vi "Umgebung.ParameterUI.vi"() -> ()   [LabVIEW 2016, in "Umgebung.lvclass"]
uses:
  Umgebung.lvclass
  Package ResourceControl/ViHandler/ViHandler.ViInfo.ctl
  Package Libraries/Message Queue/private/MessageQueue.MessageTypeDef.ctl
  Umgebung.lvclass/Umgebung.ctl
  Package ErrorHandling/ErrorHandling.lvclass/ErrorHandling.ctl
  Read Umgebung.Parameter.vi
  Package ErrorHandling/ErrorHandling.checkForErrorAndHandle.vi
  Package ErrorHandling/ErrorHandling.GetErrorHandler.vi
  Package Libraries/StringFunctions/StringFunctions_ReplaceAllBlindSigns.vi
  <vilib>/dlg_ctls.llb/Space Constant.vi
  <vilib>/Utility/error.llb/Error Cluster From Error Code.vi
  Package Libraries/TimingFunctions/TimingFunctions_getUtcTimestamp.vi
  <vilib>/Utility/error.llb/Trim Whitespace.vi
  <vilib>/Utility/error.llb/Search and Replace Pattern.vi
  Package ErrorHandling/ErrorHandling.addLastErrorToFile.vi
  <vilib>/ErrorRing/Error Ring.xnode
  Package ErrorHandling/ErrorHandling.lvclass
  Package ResourceControl/ViHandler/ViHandler.lvclass
panel:
  in  "Umgebung Parameter":T1={"Wetter"=enum."Starke Bewölkung"}
  out "Umgebung":refnum<data-value>
  in  "Model Path":path
  out "ViInfoTemp":T2
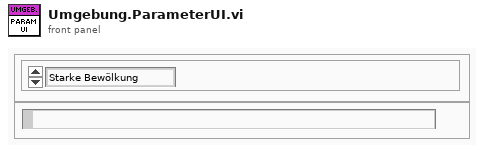
[diagram p1: front panel]
types:
  T1 = cluster{"Wetter":enum16{"Klarer Himmel", "Leichte Bewölkung", "Starke Bewölkung"}}
  T2 = typedef "ViHandler.lvclass/ViHandler.ViInfo.ctl" = cluster{"ViName":string, "ViReference":refnum<vi>, "ViQueueName":string}
  T3 = typedef "MessageQueue.MessageTypeDef.ctl" = cluster{"Message":string, "Data":variant}
  T4 = enum16{"open", "replace", "create", "open or create", "replace or create", "replace or create with confirmation"}
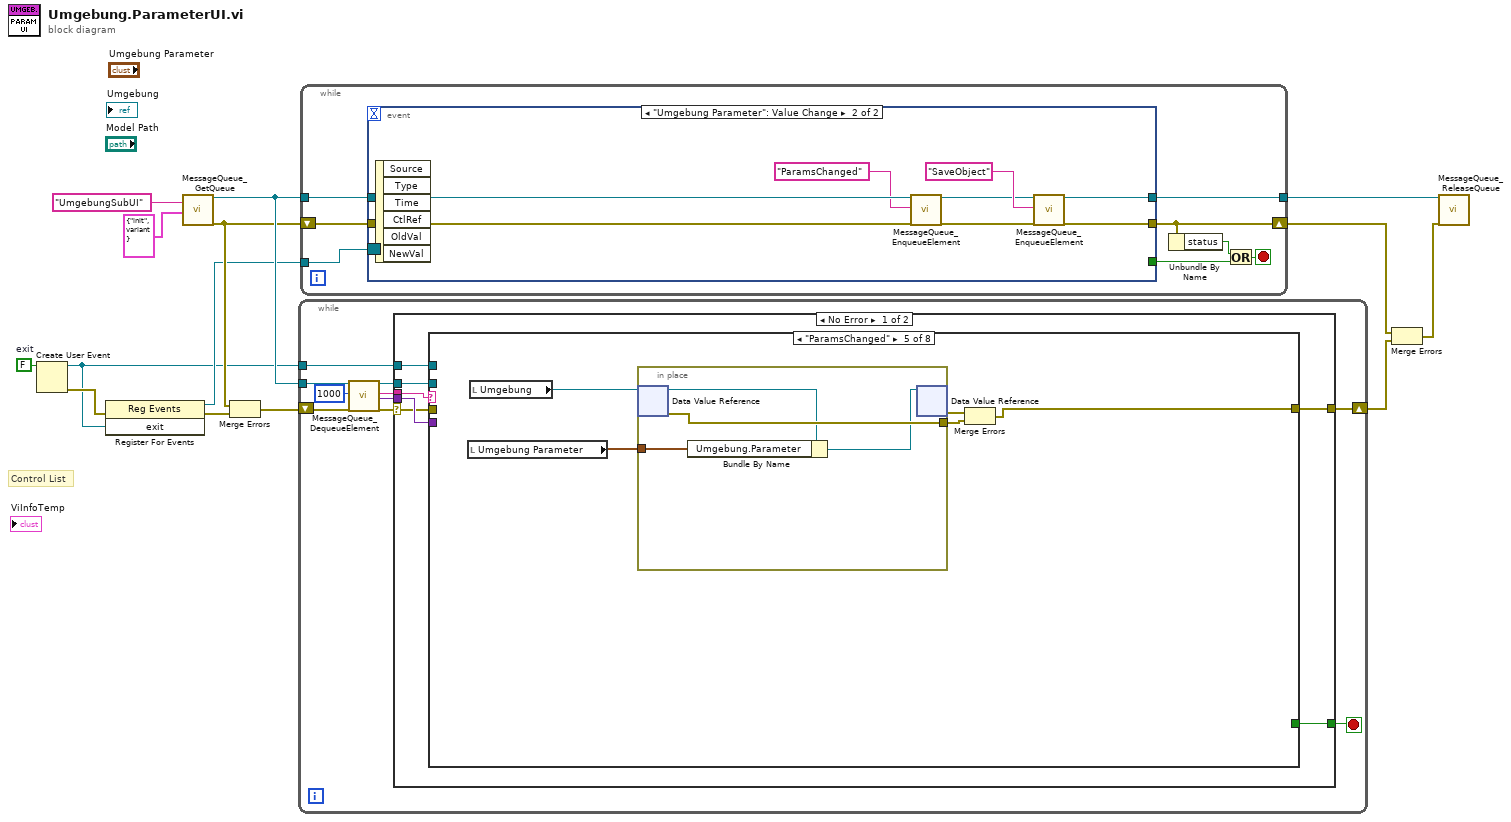
[diagram p0: block diagram]
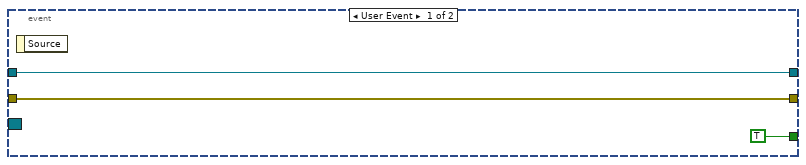
[diagram p2: hidden frame]
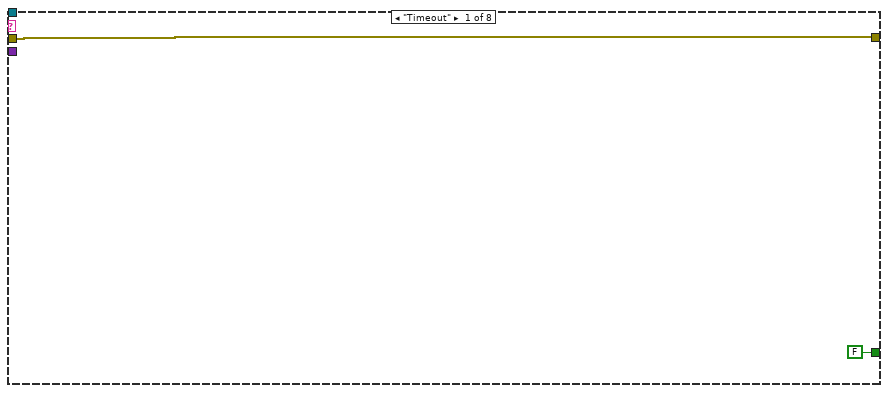
[diagram p3: hidden frame]
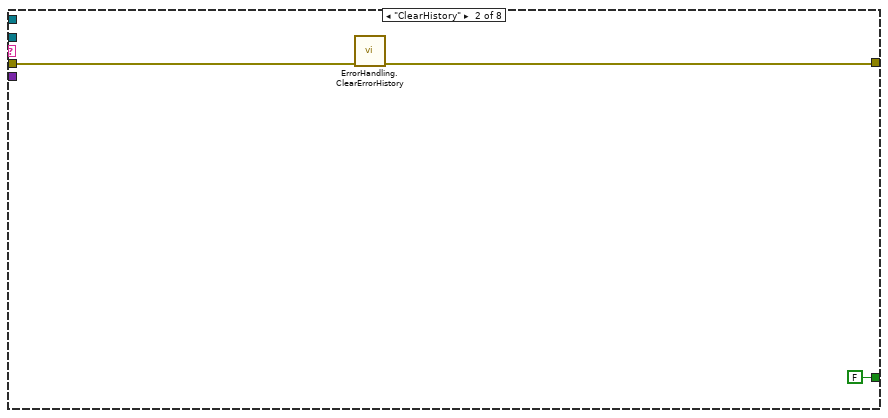
[diagram p4: hidden frame]
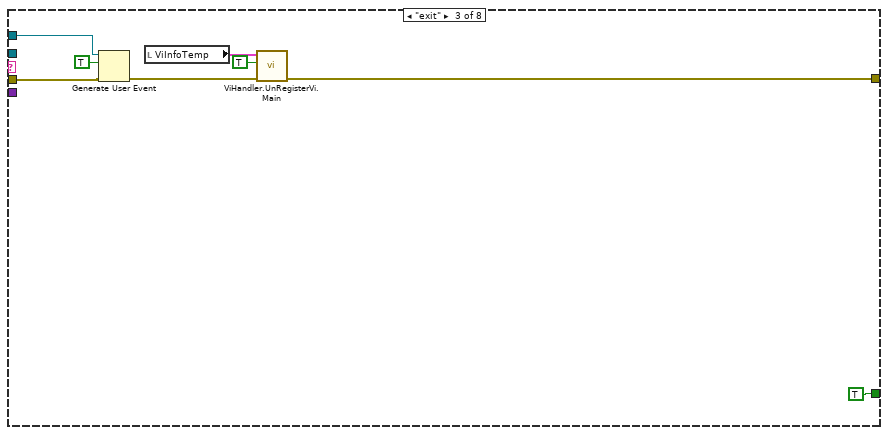
[diagram p5: hidden frame]
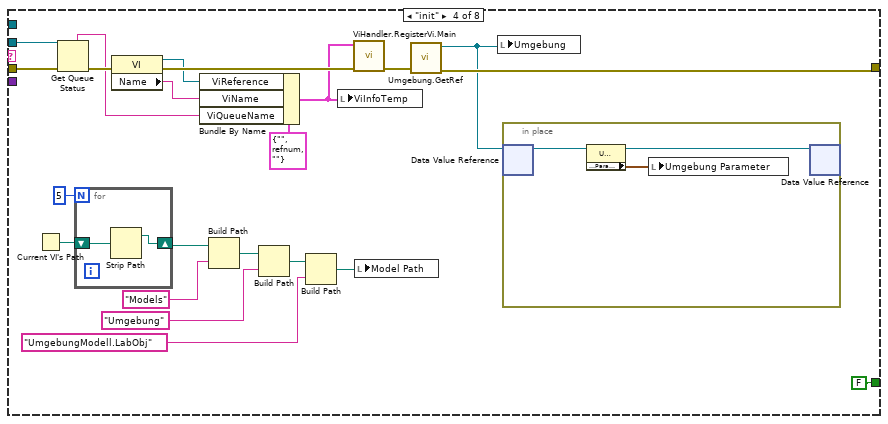
[diagram p6: hidden frame]
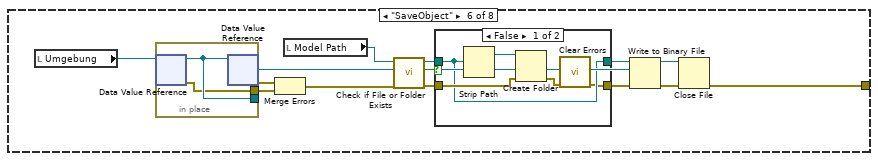
[diagram p7: hidden frame]
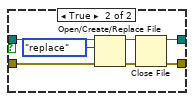
[diagram p8: hidden frame]
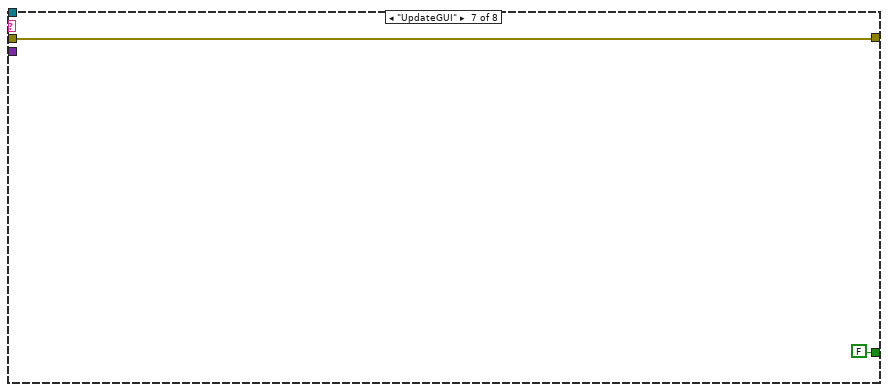
[diagram p9: hidden frame]
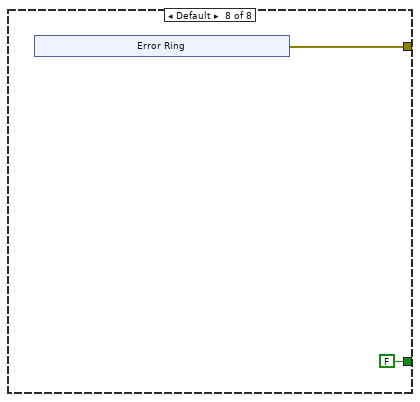
[diagram p10: hidden frame]
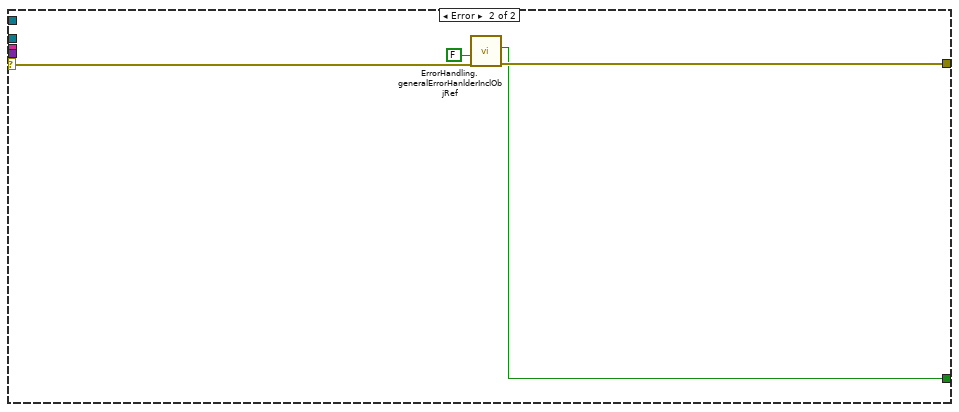
[diagram p11: hidden frame]
diagram:
  w7 = FALSE  # exit
  # "Control List"
  n1 = Create User Event(user event datatype=w7) -> (user event=w5:refnum<user-event>, error out=w6:errorcluster)  [unwired: 1 in]
  n2 = register-events(error in=w6, w5) -> (reference out=w9:refnum<event-registration>, error out=w11:errorcluster)  [unwired: 1 in]
  n3 = call "MessageQueue_GetQueue.vi"("Name"="UmgebungSubUI", "OptionalInitValue"=T3 {"Message"="init", "Data"=variant}) -> ("QueueOut"=w13:refnum<queue>, "ErrorOut"=w10:errorcluster)  [unwired: 15 in, 1 out]
  n4 = Merge Errors(w10, w11) -> (w8:errorcluster)
  n5 = while {
    tunnel: w13 -> [w24]
    tunnel: w5 -> [w17]
    shift-right: [w16] -> w3
    shift-left: w8 -> [w18]
    stop <- w19 stop-if-true
    n6 = call "MessageQueue_DequeueElement.vi"("QueueIn"=w24, "Timeout"=1000, "ErrorIn"=w18) -> ("QueueOut"=w22:refnum<queue>, "Message"=w21:string, "Data"=w20:variant, "ErrorOut"=w23:errorcluster)  [unwired: 12 in, 1 out]
    n7 = case shown="No Error" w23 {
      selector: w23 -> [w27 w121]
      tunnel: w22 -> [w31 _]
      tunnel: w21 -> [w30 _]
      tunnel: w20 -> [w29 _]
      tunnel: [w28 w119] -> w19
      tunnel: w17 -> [w26 _]
      tunnel: [w25 w120] -> w16
      frame No Error {
        n8 = case shown="\"ParamsChanged\"" w30 {
          tunnel: w31 -> [_ _ _ w60 _ _ _ _]
          tunnel: w29 -> [_ _ _ _ _ _ _ _]
          tunnel: [FALSE FALSE TRUE FALSE _ _ FALSE FALSE] -> w28
          tunnel: w27 -> [w32 w35 w42 w57 _ _ w109 _]
          tunnel: w26 -> [_ _ w41 _ _ _ _ _]
          tunnel: [w32 w34 w38 w46 w73 w82 w109 w112] -> w25
          frame "Timeout" {
          }
          frame "ClearHistory" {
            n9 = call "ErrorHandling.ClearErrorHistory.vi"("error IO"=w35) -> ("error IO"=w34:errorcluster)  [unwired: 10 in]
          }
          frame "exit" {
            n10 = Generate User Event(user event=w41, event data cluster=TRUE ("event data"), error in=w42) -> (error out=w39:errorcluster)  [unwired: 1 in, 1 out]
            n11 = local read "ViInfoTemp"() -> (w40:T2)
            n12 = call "ViHandler.UnRegisterVi.Main.vi"("ErrorIn"=w39, "FinalExit?"=TRUE, "ViInfo"=w40) -> ("ErrorOut"=w38:errorcluster)  [unwired: 7 in, 1 out]
          }
          frame "init" {
            n13 = Current VI's Path() -> (path=w48:path)
            n14 = Get Queue Status(queue=w60, error in (no error)=w57) -> (queue name=w58:string, error out=w64:errorcluster)  [unwired: 1 in, 6 out]
            n15 = for {
              N: 5 -> [_]
              shift-right: [w67] -> w55
              shift-left: w48 -> [w68]
              n16 = Strip Path(path=w68) -> (stripped path=w67:path)  [unwired: 1 out]
            }
            n17 = property class="VI"(error in=w64) -> (reference out=w62:refnum<vi>, error out=w63:errorcluster, "Name"=w61:string)  [unwired: 1 in]
            n18 = Bundle By Name(cluster=T2 {"ViName"="", "ViReference"=refnum, "ViQueueName"=""} ("ViInfo"), "ViReference"=w62, "ViName"=w61, "ViQueueName"=w58) -> (w59:T2)
            n19 = Build Path(base path=w55, name or relative path="Models") -> (appended path=w53:path)
            n20 = Build Path(base path=w53, name or relative path="Umgebung") -> (appended path=w51:path)
            n21 = Build Path(base path=w51, name or relative path="UmgebungModell.LabObj") -> (appended path=w50:path)
            n22 = local write "ViInfoTemp"(w59) -> ()
            n23 = call "ViHandler.RegisterVi.Main.vi"("ErrorIn"=w63, "ViInfo"=w59) -> ("ErrorOut"=w47:errorcluster)  [unwired: 9 in]
            n24 = local write "Model Path"(w50) -> ()
            n25 = call "Umgebung.GetRef.vi"("Error in"=w47) -> ("Error out"=w46:errorcluster, "Umgebung"=w45:refnum<data-value>)  [unwired: 9 in]
            n26 = local write "Umgebung"(w45) -> ()
            n27 = in-place {
              n28 = in-place-dvr #1(w45) -> (w71:refnum<class "Umgebung.lvclass">)  [unwired: 1 out]
              n29 = property class="Umgebung.lvclass"(reference=w71) -> (reference out=w70:refnum<class "Umgebung.lvclass">, "Accessors:Umgebung.Parameter"=w69:T1)  [unwired: 1 in, 1 out]
              n30 = local write "Umgebung Parameter"(w69) -> ()
              n31 = in-place-dvr #1(w70) -> ()  [unwired: 2 out]
            }
          }
          frame "ParamsChanged" {
            n32 = local read "Umgebung Parameter"() -> (w76:T1)
            n33 = local read "Umgebung"() -> (w72:refnum<data-value>)
            n34 = in-place {
              in-place-border: w76 -> [w77]
              in-place-border: [w80] -> w74
              n35 = in-place-dvr #2(w72) -> (w79:refnum<class "Umgebung.lvclass">, w80:errorcluster)
              n36 = Bundle By Name(cluster=w79, "Umgebung.Parameter"=w77) -> (w78:refnum<class "Umgebung.lvclass">)
              n37 = in-place-dvr #2(w78) -> (w75:errorcluster)  [unwired: 1 out]
            }
            n38 = Merge Errors(w75, w74) -> (w73:errorcluster)
          }
          frame "SaveObject" {
            n39 = local read "Umgebung"() -> (w81:refnum<data-value>)
            n40 = in-place {
              in-place-border: [w108] -> w88
              in-place-border: [w107] -> w86
              n41 = in-place-dvr #3(w81) -> (w108:refnum<class "Umgebung.lvclass">, w107:errorcluster)
              n42 = in-place-dvr #3(w108) -> (w87:errorcluster)  [unwired: 1 out]
            }
            n43 = Merge Errors(w87, w86) -> (w85:errorcluster)
            n44 = local read "Model Path"() -> (w94:path)
            n45 = call <vilib>:"Check if File or Folder Exists.vi"("error in (no error)"=w85, "path"=w94) -> ("error out"=w91:errorcluster, "file or folder exists?"=w93:bool, "dup path"=w92:path)  [unwired: 7 in]
            n46 = case shown="False" w93 {
              tunnel: w92 -> [w97 w106]
              tunnel: [w97 w102] -> w90
              tunnel: w91 -> [w98 w105]
              tunnel: [w95 w101] -> w89
              frame False {
                n47 = Strip Path(path=w97) -> (stripped path=w99:path)  [unwired: 1 out]
                n48 = Create Folder(path (use dialog)=w99, error in=w98) -> (error out=w96:errorcluster)  [unwired: 1 in, 2 out]
                n49 = call <vilib>:"Clear Errors.vi"("error in (no error)"=w96) -> ("error out"=w95:errorcluster)  [unwired: 5 in, 1 out]
              }
              frame True {
                n50 = Open/Create/Replace File(file path (use dialog)=w106, error in=w105, operation (0:open)=T4."replace") -> (refnum out=w103:refnum<file>, error out=w100:errorcluster)  [unwired: 3 in, 1 out]
                n51 = Close File(refnum=w103, error in=w100) -> (path=w102:path, error out=w101:errorcluster)
              }
            }
            n52 = Write to Binary File(file (use dialog)=w90, data=w88, error in=w89) -> (refnum out=w83:refnum<file>, error out=w84:errorcluster)  [unwired: 3 in, 1 out]
            n53 = Close File(refnum=w83, error in=w84) -> (error out=w82:errorcluster)  [unwired: 1 out]
          }
          frame "UpdateGUI" {
          }
          frame Default {
            n54 = xnode "Error Ring"() -> ("error out"=w112:errorcluster)
          }
        }
      }
      frame Error {
        n55 = call "ErrorHandling.generalErrorHanlderInclObjRef.vi"("error in"=w121, "StopOnError"=FALSE) -> ("error out"=w120:errorcluster, "Stop"=w119:bool)  [unwired: 7 in, 1 out]
      }
    }
  }
  n56 = while {
    tunnel: w13 -> [w129]
    tunnel: [w128] -> w14
    shift-right: [w125] -> w2
    shift-left: w10 -> [w127]
    tunnel: w9 -> [w122]
    stop <- w124 stop-if-true
    n57 = event shown="[1] \"Umgebung Parameter\": Value Change" {
      selector: w122 -> [_ _]
      dyn-events: _ -> [_ _]
      timeout: _ -> [_ _]
      tunnel: w129 -> [w131 w140]
      tunnel: [w131 w134] -> w128
      tunnel: [w130 w133] -> w125
      tunnel: w127 -> [w130 w139]
      tunnel: [TRUE _] -> w126
      event User Event {
        n58 = event-data() -> ()  [unwired: 1 in, 1 out]
      }
      event "Umgebung Parameter": Value Change {
        n59 = event-data() -> ()  [unwired: 1 in, 6 out]
        n60 = call "MessageQueue_EnqueueElement.vi"("QueueIn"=w140, "Message"="ParamsChanged", "ErrorIn"=w139) -> ("QueueOut"=w136:refnum<queue>, "ErrorOut"=w135:errorcluster)  [unwired: 15 in]
        n61 = call "MessageQueue_EnqueueElement.vi"("QueueIn"=w136, "Message"="SaveObject", "ErrorIn"=w135) -> ("QueueOut"=w134:refnum<queue>, "ErrorOut"=w133:errorcluster)  [unwired: 15 in]
      }
    }
    n62 = Unbundle By Name(w125) -> ("status"=w123:bool)
    n63 = Or(x=w123, y=w126) -> (x .or. y?=w124:bool)
  }
  n64 = Merge Errors(w2, w3) -> (w1:errorcluster)
  n65 = call "MessageQueue_ReleaseQueue.vi"("QueueIn"=w14, "ErrorIn"=w1) -> ()  [unwired: 15 in, 3 out]
